vi "unset tag writer or reader.vi"(7 "module GUID":string, 8 "error in":errorcluster, 9 "channel":refnum<class "TBM channel.lvclass">, 10 "tag descriptor":refnum<class "tag descriptor.lvclass">, 11 "engine configuration in":refnum<class "engine configuration.lvclass">) -> (0 "error out":errorcluster, 3 "engine configuration out":refnum<class "engine configuration.lvclass">)   [LabVIEW 2013, in "engine configuration.lvclass"]
uses:
  engine configuration.lvclass
  <vilib>/NI/Tag Bus/tag/tag descriptor.lvclass
  <vilib>/NI/Tag Bus Module Framework/channel/TBM channel.lvclass
  <vilib>/NI/Tag Bus/tag/tag descriptor.lvclass/tag descriptor.ctl
  <vilib>/NI/Tag Bus Module Framework/channel/TBM channel.lvclass/TBM channel.ctl
  engine configuration.lvclass/engine configuration.ctl
  <vilib>/NI/Tag Bus/tag/read tag name.vi
  <vilib>/NI/Tag Bus Module Framework/channel/Read channel classification.vi
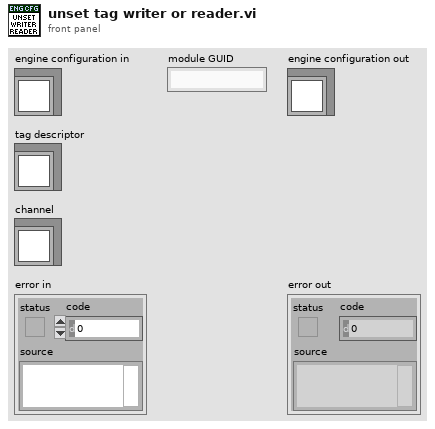
[diagram p1: front panel]
types:
  T1 = typedef "TBM channel.lvclass/channel classification.ctl" = enum16{"input data", "output data", "processing parameter", "processing result"}
  T2 = typedef "engine configuration.lvclass/module channel pairings.ctl" = cluster{"modules":string[], "channels":string[]}
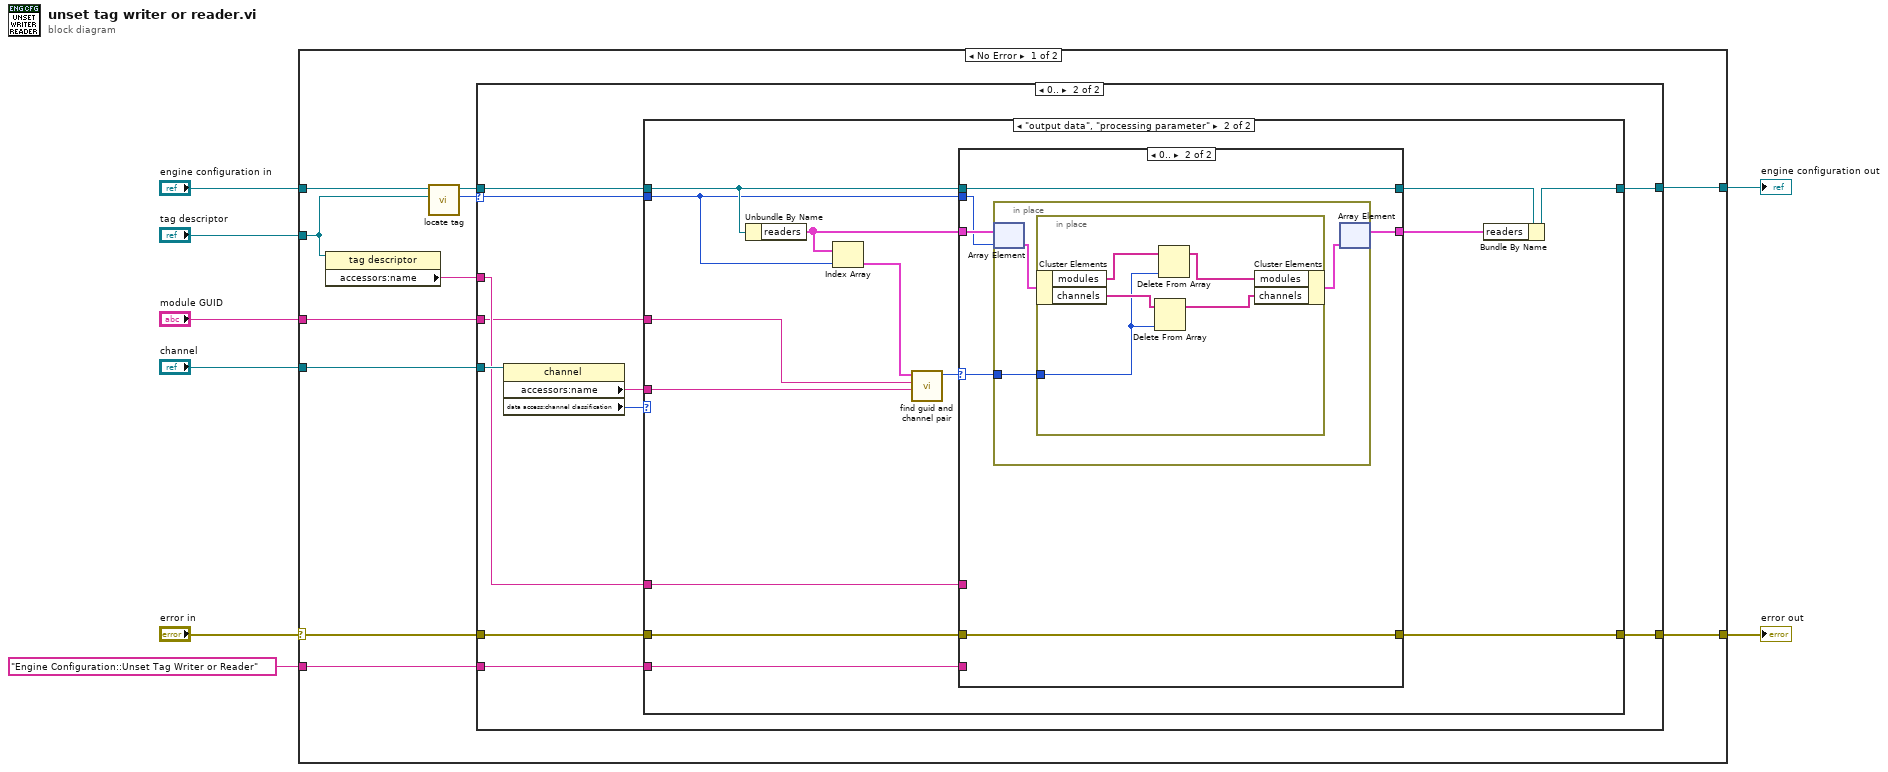
[diagram p0: block diagram]
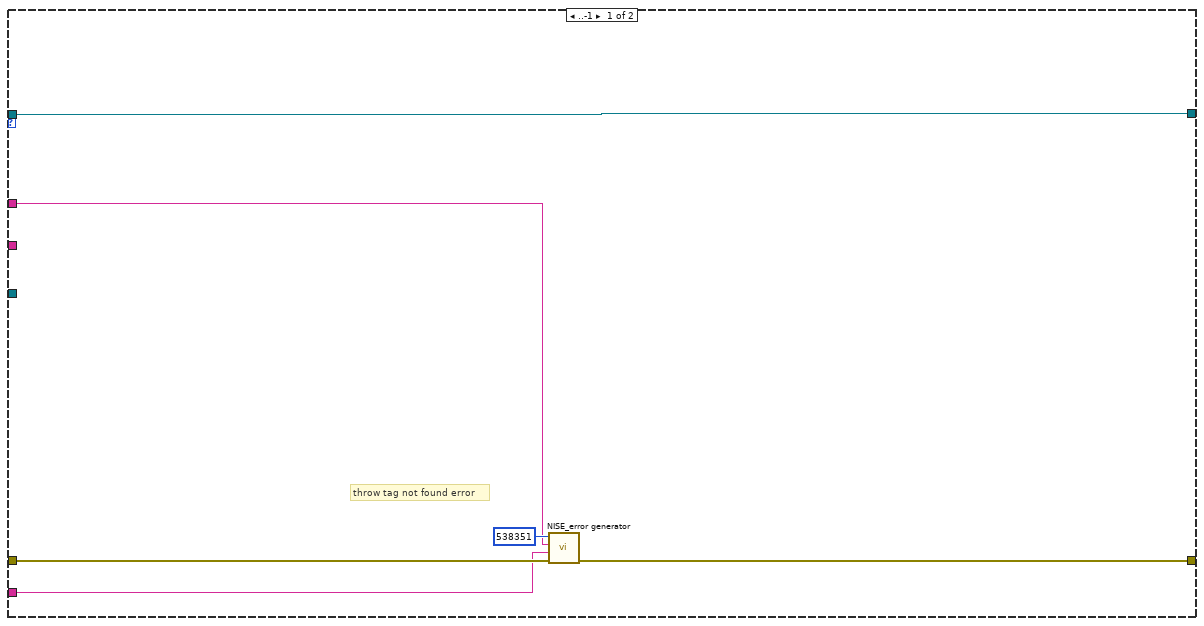
[diagram p2: hidden frame]
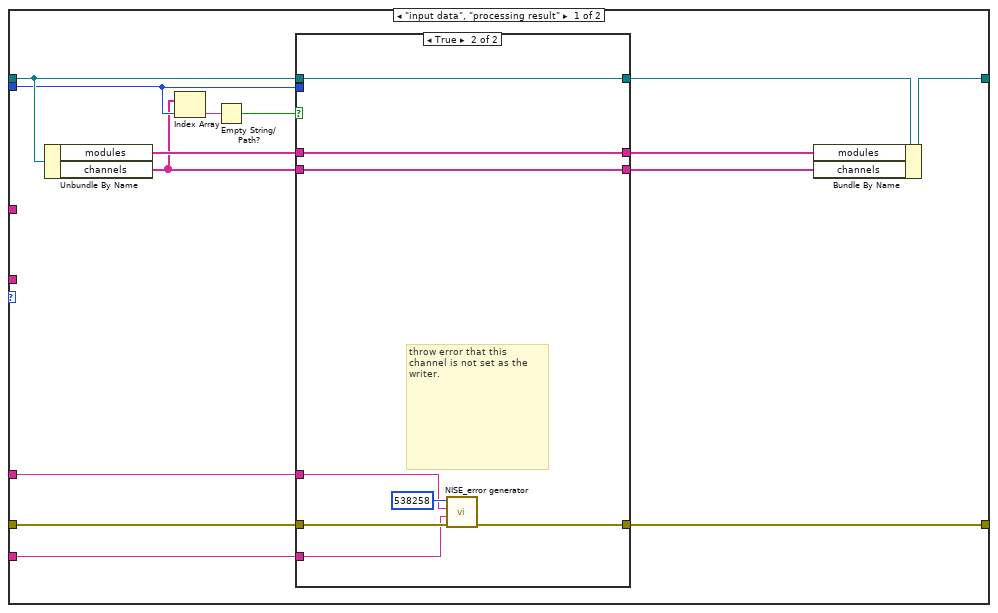
[diagram p3: hidden frame]
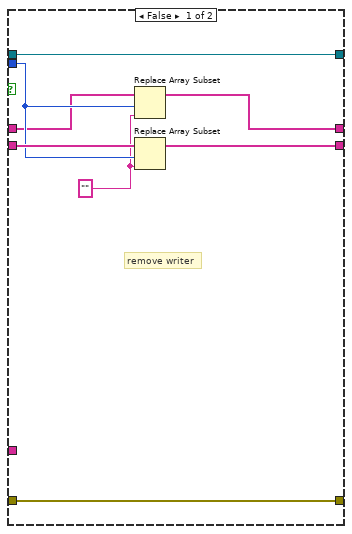
[diagram p4: hidden frame]
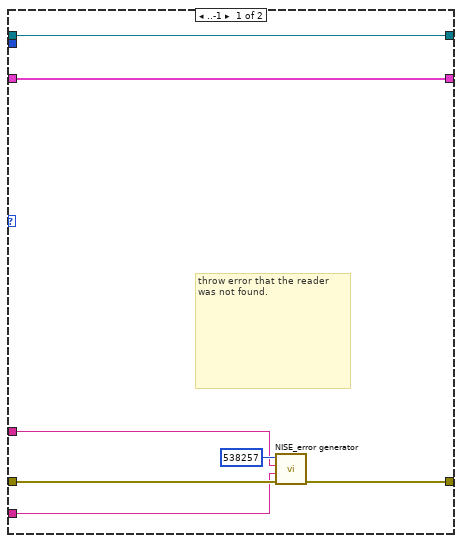
[diagram p5: hidden frame]
diagram:
  n1 = case shown="No Error" "error in" {
    selector: "error in" -> [w15 w103]
    tunnel: [w13 w103] -> w7
    tunnel: [w12 w102] -> w5
    tunnel: "engine configuration in" -> [w19 w102]
    tunnel: "tag descriptor" -> [w11 _]
    tunnel: "module GUID" -> [w16 _]
    tunnel: "channel" -> [w17 _]
    tunnel: "Engine Configuration::Unset Tag Writer or Reader" ("source") -> [w9 _]
    frame No Error {
      n2 = property class="tag descriptor"(reference=w11) -> ("accessors:name"=w10:string)  [unwired: 1 in, 2 out]
      n3 = call "locate tag.vi"("tag descriptor"=w11, "engine configuration in"=w19) -> ("index"=w14:i32, "engine configuration out"=w18:refnum<class "engine configuration.lvclass">)  [unwired: 8 in]
      n4 = case shown="0.." w14 {
        selector: w14 -> [_ w34]
        tunnel: w18 -> [w25 w33]
        tunnel: w17 -> [_ w36]
        tunnel: w16 -> [_ w26]
        tunnel: w15 -> [w23 w35]
        tunnel: [w22 w32] -> w13
        tunnel: [w25 w28] -> w12
        tunnel: w10 -> [w21 w30]
        tunnel: w9 -> [w20 w31]
        frame ..-1 {
          # "throw tag not found error"
          n5 = call <vilib>:"NISE_error generator.vi"("error in"=w23, "source"=w20, "append error message"=w21, "error code (0)"=538351) -> ("error out"=w22:errorcluster)  [unwired: 5 in]
        }
        frame 0.. {
          n6 = property class="channel"(reference=w36) -> ("accessors:name"=w27:string, "data access:channel classification"=w29:T1)  [unwired: 1 in, 2 out]
          n7 = case shown="\"output data\", \"processing parameter\"" w29 {
            tunnel: w35 -> [w50 w79]
            tunnel: w34 -> [w42 w69]
            tunnel: w33 -> [w44 w74]
            tunnel: [w43 w73] -> w28
            tunnel: [w48 w78] -> w32
            tunnel: w31 -> [w47 w76]
            tunnel: w30 -> [w46 w77]
            tunnel: w27 -> [_ w67]
            tunnel: w26 -> [_ w68]
            frame "input data", "processing result" {
              n8 = Unbundle By Name(w44) -> ("modules"=w40:string[], "channels"=w39:string[])
              n9 = Index Array(array=w39, index=w42) -> (element=w45:string)
              n10 = Empty String/Path?(string/path=w45) -> (empty?=w41:bool)
              n11 = case shown="True" w41 {
                tunnel: w50 -> [w58 w64]
                tunnel: [w58 w63] -> w48
                tunnel: w44 -> [w57 w66]
                tunnel: [w57 w66] -> w49
                tunnel: w42 -> [w55 _]
                tunnel: w47 -> [_ w62]
                tunnel: w46 -> [_ w61]
                tunnel: w40 -> [w54 w60]
                tunnel: w39 -> [w56 w59]
                tunnel: [w53 w60] -> w38
                tunnel: [w52 w59] -> w37
                frame False {
                  w51 = "" ("new element/subarray")
                  # "remove writer"
                  n12 = Replace Array Subset(array=w54, new element=w51, index=w55) -> (w53:string[])
                  n13 = Replace Array Subset(array=w56, new element=w51, index=w55) -> (w52:string[])
                }
                frame True {
                  # "throw error that this channel is not set as the writer."
                  n14 = call <vilib>:"NISE_error generator.vi"("error in"=w64, "source"=w62, "append error message"=w61, "error code (0)"=538258) -> ("error out"=w63:errorcluster)  [unwired: 5 in]
                }
              }
              n15 = Bundle By Name(cluster=w49, "modules"=w38, "channels"=w37) -> (w43:refnum<class "engine configuration.lvclass">)
            }
            frame "output data", "processing parameter" {
              n16 = Unbundle By Name(w74) -> ("readers"=w71:T2[])
              n17 = Index Array(array=w71, index=w69) -> (element=w75:T2)
              n18 = call "find guid and channel pair.vi"("channel name"=w67, "Module GUID"=w68, "listing"=w75) -> ("index"=w70:i32)  [unwired: 8 in]
              n19 = case shown="0.." w70 {
                selector: w70 -> [_ w88]
                tunnel: w74 -> [w87 w93]
                tunnel: [w87 w93] -> w80
                tunnel: w79 -> [w85 w92]
                tunnel: [w84 w92] -> w78
                tunnel: w77 -> [w83 _]
                tunnel: w76 -> [w82 _]
                tunnel: [w81 w89] -> w72
                tunnel: w71 -> [w81 w91]
                tunnel: w69 -> [_ w90]
                frame ..-1 {
                  # "throw error that the reader was not found."
                  n20 = call <vilib>:"NISE_error generator.vi"("error in"=w85, "source"=w82, "append error message"=w83, "error code (0)"=538257) -> ("error out"=w84:errorcluster)  [unwired: 5 in]
                }
                frame 0.. {
                  n21 = in-place {
                    in-place-border: w88 -> [w94]
                    n22 = in-place-array #1(w91, w90) -> (w96:T2)
                    n23 = in-place {
                      in-place-border: w94 -> [w97]
                      n24 = in-place-cluster #2(w96) -> ("modules"=w101:string[], "channels"=w99:string[])
                      n25 = Delete From Array(array=w99, index=w97) -> (array with subset deleted=w98:string[])  [unwired: 1 in, 1 out]
                      n26 = Delete From Array(array=w101, index=w97) -> (array with subset deleted=w100:string[])  [unwired: 1 in, 1 out]
                      n27 = in-place-cluster #2("modules"=w100, "channels"=w98) -> (w95:T2)
                    }
                    n28 = in-place-array #1(w95) -> (w89:T2[])  [unwired: 1 out]
                  }
                }
              }
              n29 = Bundle By Name(cluster=w80, "readers"=w72) -> (w73:refnum<class "engine configuration.lvclass">)
            }
          }
        }
      }
    }
    frame Error {
    }
  }
  "error out" <- w7
  "engine configuration out" <- w5
